vi "SetSP_State.vi"(8 "error in (no error)":errorcluster, 9 "Ancestor":string, 10 "SP Open":bool, 11 "reference in":refnum<class "ViPER.lvclass">) -> (0 "error out":errorcluster, 3 "reference out":refnum<class "ViPER.lvclass">)   [LabVIEW 2022 SP3, in "ViPER.lvlib" / "ViPER.lvclass"]
doc: "### BSD License (http://www.opensource.org/licenses/bsd-license.php) Begin ###\n\nCopyright (c) 2018 Kurt Friday www.medulla.net\n\nAll rights reserved.\n\nRedistribution and use in source and binary forms, with or without\nmodification, are permitted provided that the following conditions are met:\n\n * Redistributions of source code must retain the above copyright\n notice, this list of conditions and the following disclaimer.\n\n * Redistributions in binary form must reproduce the above copyright\n notice, this list of conditions and the following disclaimer in the\n documentation and/or other materials provided with the distribution.\n\n * Neither the name of the <organization> nor the\n names of its contributors may be used to endorse or promote products\n derived from this software without specific prior written permission.\n\nTHIS SOFTWARE IS PROVIDED BY THE COPYRIGHT HOLDERS AND CONTRIBUTORS \"AS IS\" AND\nANY EXPRESS OR IMPLIED WARRANTIES, INCLUDING, BUT NOT LIMITED TO, THE IMPLIED\nWARRANTIES OF MERCHANTABILITY AND FITNESS FOR A PARTICULAR PURPOSE ARE\nDISCLAIMED. IN NO EVENT SHALL <COPYRIGHT HOLDER> BE LIABLE FOR ANY\nDIRECT, INDIRECT, INCIDENTAL, SPECIAL, EXEMPLARY, OR CONSEQUENTIAL DAMAGES\n(INCLUDING, BUT NOT LIMITED TO, PROCUREMENT OF SUBSTITUTE GOODS OR SERVICES;\nLOSS OF USE, DATA, OR PROFITS; OR BUSINESS INTERRUPTION) HOWEVER CAUSED AND\nON ANY THEORY OF LIABILITY, WHETHER IN CONTRACT, STRICT LIABILITY, OR TORT\n(INCLUDING NEGLIGENCE OR OTHERWISE) ARISING IN ANY WAY OUT OF THE USE OF THIS\nSOFTWARE, EVEN IF ADVISED OF THE POSSIBILITY OF SUCH DAMAGE."
uses:
  ViPER.lvclass
panel:
  # "### BSD License (http://www.opensource.org/licenses/bsd-license.php) Begin ###\n\nCopyright (c) 2018  Kurt Friday www.medulla.net\n\nAll rights reserved.\n\nRedistribution and use in source and binary forms, with or without\nmodification, are permitted provided that the following conditions are met:\n\n    * Redistributions of source code must retain the above copyright\n      notice, this list of conditions and the following disclaimer.\n\n    * Redistributions in binary form must reproduce the above copyright\n      notice, this list of conditions and the following disclaimer in the\n      documentation and/or other materials provided with the distribution.\n\n    * Neither the name of the <organization> nor the\n      names of its contributors may be used to endorse or promote products\n      derived from this software without specific prior written permission.\n\nTHIS SOFTWARE IS PROVIDED BY THE COPYRIGHT HOLDERS AND CONTRIBUTORS \"AS IS\" AND\nANY EXPRESS OR IMPLIED WARRANTIES, INCLUDING, BUT NOT LIMITED TO, THE IMPLIED\nWARRANTIES OF MERCHANTABILITY AND FITNESS FOR A PARTICULAR PURPOSE ARE\nDISCLAIMED. IN NO EVENT SHALL <COPYRIGHT HOLDER> BE LIABLE FOR ANY\nDIRECT, INDIRECT, INCIDENTAL, SPECIAL, EXEMPLARY, OR CONSEQUENTIAL DAMAGES\n(INCLUDING, BUT NOT LIMITED TO, PROCUREMENT OF SUBSTITUTE GOODS OR SERVICES;\nLOSS OF USE, DATA, OR PROFITS; OR BUSINESS INTERRUPTION) HOWEVER CAUSED AND\nON ANY THEORY OF LIABILITY, WHETHER IN CONTRACT, STRICT LIABILITY, OR TORT\n(INCLUDING NEGLIGENCE OR OTHERWISE) ARISING IN ANY WAY OUT OF THE USE OF THIS\nSOFTWARE, EVEN IF ADVISED OF THE POSSIBILITY OF SUCH DAMAGE."
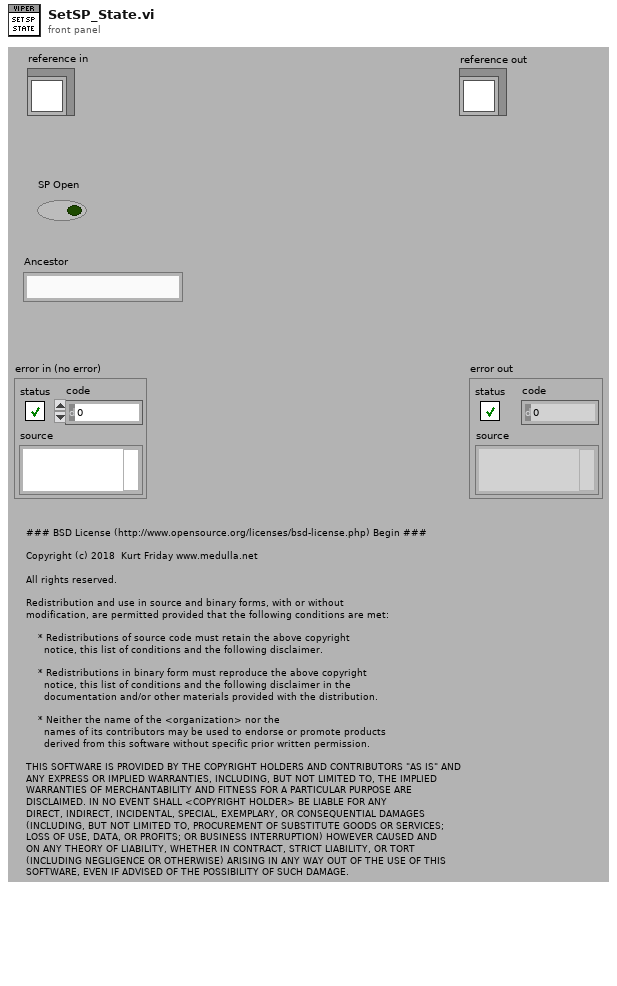
[diagram p1: front panel]
types:
  T1 = typedef "ViPER.lvlib/ViPER.lvclass/Details.ctl" = cluster{"Name":string, "Class":string}
  T2 = typedef "ViPER.lvlib/ViPER.lvclass/ObjectAttributes.ctl" = cluster{"Object":T3, "Ancestors":T5[], "Config":T6, "Init_OK":bool, "Hierachy":string[], "PPL?":bool[], "SFP_Open":bool[], "Config_SFP_Open":bool[], "SoftFP_event":refnum<user-event>[], "ConfigFP_event":refnum<user-event>[], "SoftFP_Shutdown_Notifier":refnum<notifier>[], "ConfigFP_Shutdown_Notifier":refnum<notifier>[]}
  T3 = typedef "ViPER.lvlib/ViPER.lvclass/ObjectDefinition.ctl" = cluster{"Name":string, "Ancestors":T4[]}
  T4 = typedef "ViPER.lvlib/ViPER.lvclass/Ancestor.ctl" = cluster{"Class":string, "Config":string, "Objects":string[]}
  T5 = typedef "ViPER.lvlib/ViPER.lvclass/ObjectLayers.ctl" = cluster{"Ancestor":string, "Objects":refnum<class "ViPER.lvclass">[], "Object_Names":string[], "Owned":bool[]}
  T6 = typedef "ViPER.lvlib/ViPER.lvclass/Config.ctl" = cluster{"default":string}
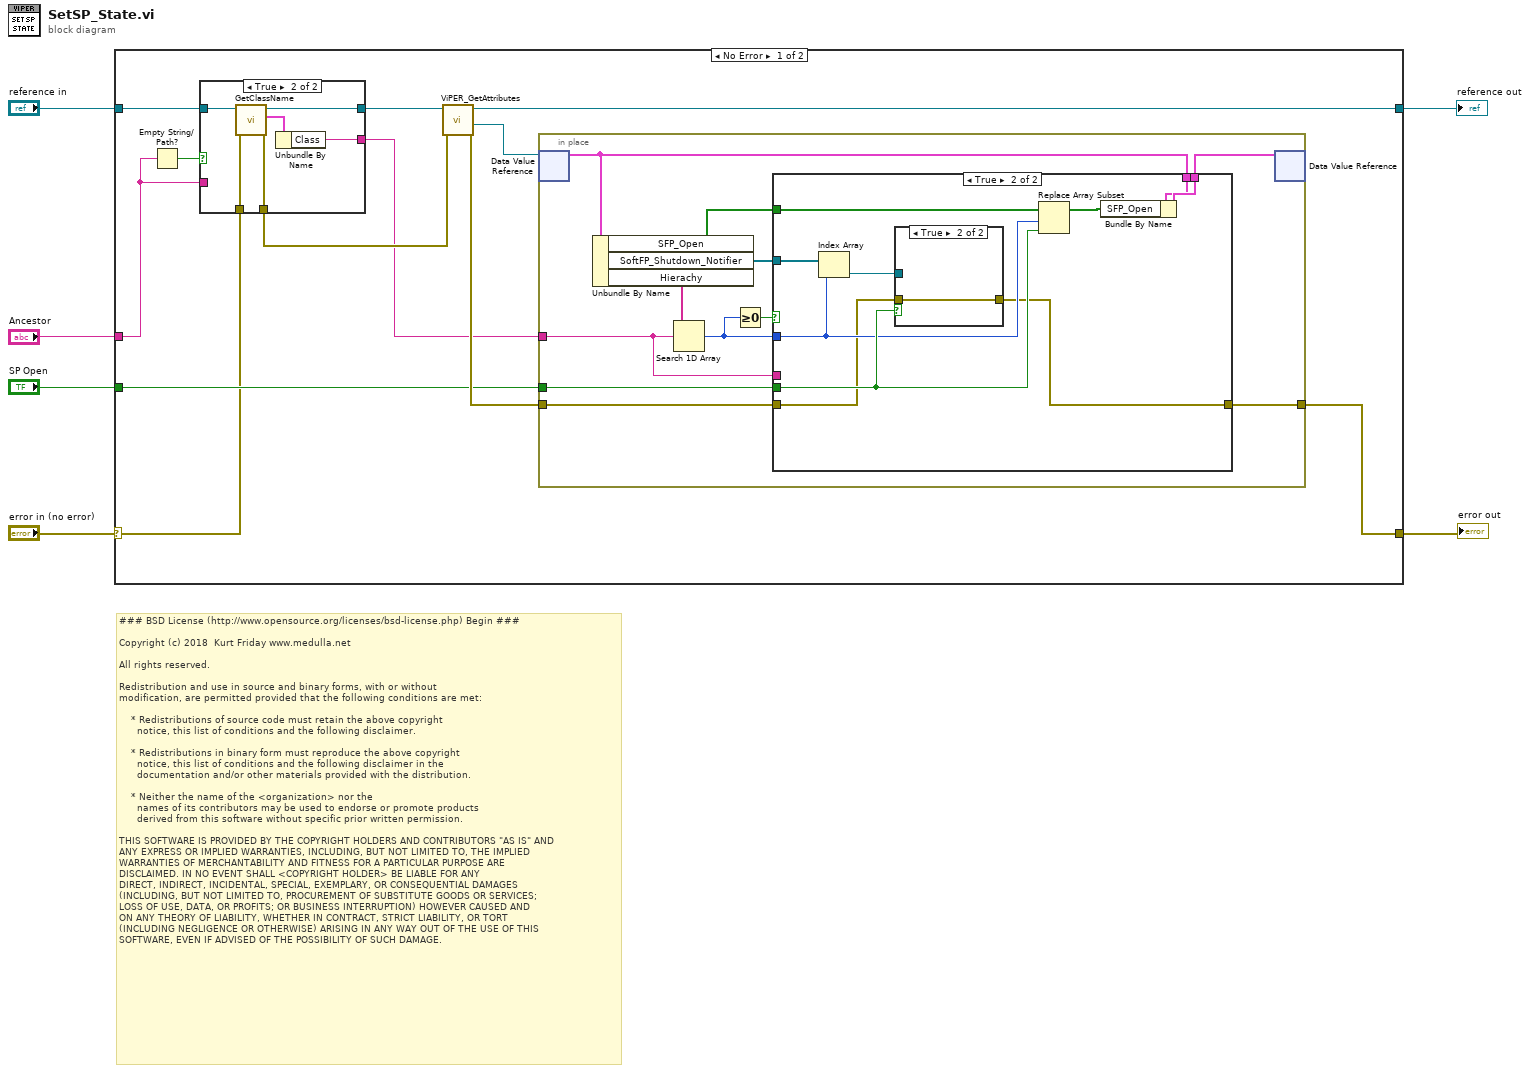
[diagram p0: block diagram]
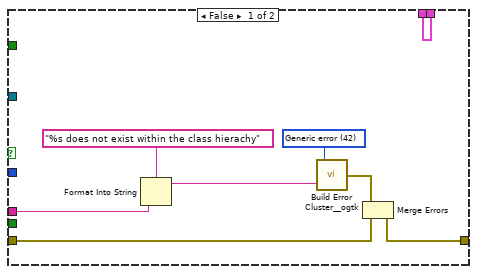
[diagram p3: hidden frame]
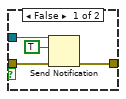
[diagram p4: hidden frame]
diagram:
  # "### BSD License (http://www.opensource.org/licenses/bsd-license.php) Begin ###\n\nCopyright (c) 2018  Kurt Friday www.medulla.net\n\nAll rights reserved.\n\nRedistribution and use in source and binary forms, with or without\nmodification, are permitted provided that the following conditions are met:\n\n    * Redistributions of source code must retain the above copyright\n      notice, this list of conditions and the following disclaimer.\n\n    * Redistributions in binary form must reproduce the above copyright\n      notice, this list of conditions and the following disclaimer in the\n      documentation and/or other materials provided with the distribution.\n\n    * Neither the name of the <organization> nor the\n      names of its contributors may be used to endorse or promote products\n      derived from this software without specific prior written permission.\n\nTHIS SOFTWARE IS PROVIDED BY THE COPYRIGHT HOLDERS AND CONTRIBUTORS \"AS IS\" AND\nANY EXPRESS OR IMPLIED WARRANTIES, INCLUDING, BUT NOT LIMITED TO, THE IMPLIED\nWARRANTIES OF MERCHANTABILITY AND FITNESS FOR A PARTICULAR PURPOSE ARE\nDISCLAIMED. IN NO EVENT SHALL <COPYRIGHT HOLDER> BE LIABLE FOR ANY\nDIRECT, INDIRECT, INCIDENTAL, SPECIAL, EXEMPLARY, OR CONSEQUENTIAL DAMAGES\n(INCLUDING, BUT NOT LIMITED TO, PROCUREMENT OF SUBSTITUTE GOODS OR SERVICES;\nLOSS OF USE, DATA, OR PROFITS; OR BUSINESS INTERRUPTION) HOWEVER CAUSED AND\nON ANY THEORY OF LIABILITY, WHETHER IN CONTRACT, STRICT LIABILITY, OR TORT\n(INCLUDING NEGLIGENCE OR OTHERWISE) ARISING IN ANY WAY OUT OF THE USE OF THIS\nSOFTWARE, EVEN IF ADVISED OF THE POSSIBILITY OF SUCH DAMAGE."
  n1 = case shown="No Error" "error in (no error)" {
    selector: "error in (no error)" -> [w11 w63]
    tunnel: [w15 w63] -> w5
    tunnel: [w18 w62] -> w3
    tunnel: "reference in" -> [w13 w62]
    tunnel: "SP Open" -> [w14 _]
    tunnel: "Ancestor" -> [w8 _]
    frame No Error {
      n2 = Empty String/Path?(string/path=w8) -> (empty?=w9:bool)
      n3 = case shown="True" w9 {
        tunnel: w11 -> [w20 w27]
        tunnel: [w20 w26] -> w10
        tunnel: w13 -> [w21 w25]
        tunnel: [w21 w24] -> w12
        tunnel: w8 -> [w19 _]
        tunnel: [w19 w22] -> w7
        frame False {
        }
        frame True {
          n4 = call "GetClassName.vi"("error in (no error)"=w27, "reference in"=w25) -> ("error out"=w26:errorcluster, "Details"=w23:T1, "reference out"=w24:refnum<class "ViPER.lvclass">)  [unwired: 7 in]
          n5 = Unbundle By Name(w23) -> ("Class"=w22:string)
        }
      }
      n6 = call "ViPER_GetAttributes.vi"("error in (no error)"=w10, "reference in"=w12) -> ("error out"=w16:errorcluster, "DataRef"=w17:refnum<data-value>, "reference out"=w18:refnum<class "ViPER.lvclass">)  [unwired: 6 in, 1 out]
      n7 = in-place {
        in-place-border: w14 -> [w33]
        in-place-border: w7 -> [w28]
        in-place-border: w16 -> [w30]
        in-place-border: [w29] -> w15
        n8 = in-place-dvr #1(w17) -> (w37:T2)  [unwired: 1 out]
        n9 = Unbundle By Name(w37) -> ("SFP_Open"=w34:bool[], "SoftFP_Shutdown_Notifier"=w35:refnum<notifier>[], "Hierachy"=w36:string[])
        n10 = Search 1D Array(1D array=w36, element=w28) -> (index of element=w32:i32)  [unwired: 1 in]
        n11 = Greater Or Equal To 0?(x=w32) -> (x >= 0?=w31:bool)
        n12 = case shown="True" w31 {
          tunnel: [w46 w56] -> w38
          tunnel: w37 -> [w46 w55]
          tunnel: w35 -> [_ w54]
          tunnel: w34 -> [_ w52]
          tunnel: w33 -> [_ w51]
          tunnel: w32 -> [_ w49]
          tunnel: w30 -> [w44 w48]
          tunnel: [w43 w47] -> w29
          tunnel: w28 -> [w40 _]
          frame False {
            w42 = 42 items=["No error", "Argument error", "Memory is full", "Out of zone", "End of file", "File already open", "Generic file I/O error", "File not found", "File permission error", "Disk is full", "Duplicate path", "Too many files open", "System feature not enabled", "Resource file not found", "Cannot add resource", "Resource not found", "Image not found", "Image memory error", "Pen does not exist", "Config type invalid", "Config token not found", "Config parse error", "Config memory error", "Bad external code format", "Bad external code offset", "External code not present", "Null window", "Destroy window error", "Null menu", "Print aborted", "Bad print record", "Print driver error", "Windows error during printing", "Memory error during printing", "Print dialog error", "Generic print error", "Invalid device refnum", "Device not found", "Device parameter error", "Device unit error", "Cannot open device", "Device call aborted", "Generic error", "Cancelled by user", "Object ID too low", "Object ID too high", "Object not in heap", "Unknown heap", "Unknown object (invalid DefProc)", "Unknown object (DefProc not in table)", "Message out of range", "Invalid (null) method", "Unknown message", "Manager call not supported", "Bad address", "Network operation in progress", "Network operation timed out", "Connection is busy", "Network attribute not supported", "Network error", "Address in use", "System out of memory", "Connection aborted", "Connection refused", "Not connected", "Already connected", "Connection closed", "Initialization error (interapplication manager)", "Bad occurrence", "Wait on unbound occurrence handler", "Occurrence queue overflow", "Datalog type conflict", "Unused", "Unrecognized type (interapplication manager)", "Memory corrupt", "Failed to make temporary DLL", "Old CIN version", "Drag socket not found", "Failed to load drop-object", "Failed to register OLE object", "Failed to release OLE object", "Format specifier type mismatch", "Unknown format specifier", "Too few format specifiers", "Too many format specifiers", "Scan failed", "Newer CIN version", "Error converting to variant", "Runtime menu error", "Password tampered", "Variant attribute not found", "Incompatible variant data type", "Event data is not available", "Event Store is not present", "Occurrence is not found", "Event Queue is not created", "Event info is not available", "Refnum passed is NULL", "Error retrieving Class GUID", "Error retrieving CoClass GUID", "Error retrieving TypeLib GUID.", "Bad built application magic bytes.", "Specific driver is different from the specific driver associated with the Logical Name.", "There is no session opened to the class driver.", "Max Error", "MAX - Error with config objects", "MAX - Error loading configuration", "MAX - Group not supported"]
            n13 = Format Into String(format string="%s does not exist within the class hierachy", w40) -> (resulting string=w39:string)  [unwired: 2 in, 1 out]
            n14 = call <userlib>:"Build Error Cluster__ogtk.vi"("String to Prepend to source (\"\")"=w39, "code"=w42) -> ("error out"=w45:errorcluster)
            n15 = Merge Errors(w45, w44) -> (w43:errorcluster)
          }
          frame True {
            n16 = Index Array(array=w54, index=w49) -> (element=w53:refnum<notifier>)
            n17 = case shown="True" w51 {
              tunnel: w53 -> [w60 _]
              tunnel: w48 -> [w58 w61]
              tunnel: [w57 w61] -> w47
              frame False {
                n18 = Send Notification(notification=TRUE, notifier=w60, error in (no error)=w58) -> (error out=w57:errorcluster)  [unwired: 1 out]
              }
              frame True {
              }
            }
            n19 = Replace Array Subset(array=w52, new element=w51, index=w49) -> (w50:bool[])
            n20 = Bundle By Name(cluster=w55, "SFP_Open"=w50) -> (w56:T2)
          }
        }
        n21 = in-place-dvr #1(w38) -> ()  [unwired: 2 out]
      }
    }
    frame Error {
    }
  }
  "error out" <- w5
  "reference out" <- w3
